vi "Do_Ramsete_SI.vi"(5 "LeftDist-Meters":dbl, 6 "WheelBase-Meters":dbl=2.0, 7 "RightDist-Meters":dbl, 8 "Ramsete Enable":bool, 9 "Path Sample":T4, 10 "Reset":bool, 11 "Gyro-Radians":dbl) -> (0 "AtReference":bool, 1 "RightVelDmd":dbl, 2 "LeftVelDmd":dbl, 3 "CurrentRelativePose":T1, 4 "Err Pose":T1)   [LabVIEW 2019, in "PathExecution_Library.lvlib"]
uses:
  PathExecution_Library.lvlib
  PATH_SAMPLE.ctl
  POSE.ctl
  TRANSLATION.ctl
  ROTATION.ctl
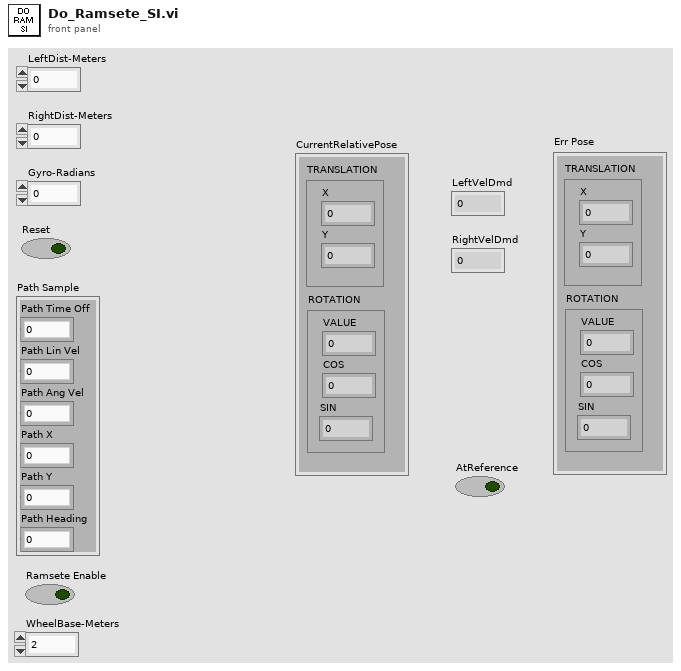
[diagram p1: front panel]
types:
  T1 = typedef "PathExecution_Library.lvlib/POSE.ctl" = cluster{"TRANSLATION":T2, "ROTATION":T3}
  T2 = typedef "PathExecution_Library.lvlib/TRANSLATION.ctl" = cluster{"X":dbl, "Y":dbl}
  T3 = typedef "PathExecution_Library.lvlib/ROTATION.ctl" = cluster{"VALUE":dbl, "COS":dbl, "SIN":dbl}
  T4 = typedef "PathExecution_Library.lvlib/PATH_SAMPLE.ctl" = cluster{"Path Lin Vel":dbl, "Path Ang Vel":dbl, "Path X":dbl, "Path Y":dbl, "Path Heading":dbl, "Path Time Off":dbl}
  T5 = typedef "PathExecution_Library.lvlib/CHASSIS.ctl" = cluster{"vX":dbl, "vY":dbl, "vOmega":dbl}
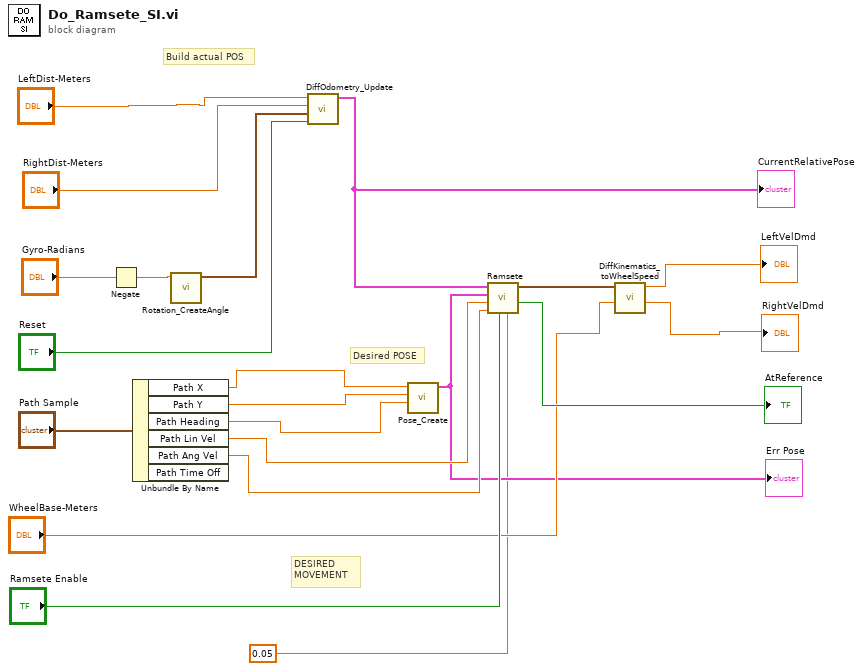
[diagram p0: block diagram]
diagram:
  # "DESIRED\nMOVEMENT"
  # "Desired POSE"
  # "Build actual POS"
  n1 = Negate(x="Gyro-Radians") -> (-x=w3:dbl)
  n2 = Unbundle By Name("Path Sample") -> ("Path X"=w13:dbl, "Path Y"=w12:dbl, "Path Heading"=w11:dbl, "Path Lin Vel"=w10:dbl, "Path Ang Vel"=w9:dbl)  [unwired: 1 out]
  n3 = call "Rotation_CreateAngle.vi"("Angle"=w3) -> ("ROTATION"=w2:T3)  [unwired: 10 in]
  n4 = call "DiffOdometry_Update.vi"("Reset"="Reset", "Heading"=w2, "RightDistance"="RightDist-Meters", "LeftDistance"="LeftDist-Meters") -> ("CurrentRelativePose"=w18:T1)  [unwired: 7 in]
  "CurrentRelativePose" <- w18
  n5 = call "Pose_Create.vi"("Heading"=w11, "Y"=w12, "X"=w13) -> ("out POSe"=w5:T1)  [unwired: 8 in]
  "Err Pose" <- w5
  n6 = call "Ramsete.vi"("POSE TOL"=0.05, "Enabled"="Ramsete Enable", "DesiredAngularVelocity"=w9, "DesiredLinearVelocity"=w10, "DesiredPOSE"=w5, "CurrentPOSE"=w18) -> ("AtReference"=→"AtReference":bool, "CHASSIS Speeds"=w16:T5)  [unwired: 3 in, 1 out]
  n7 = call "DiffKinematics_toWheelSpeed.vi"("TrackWidth_Meters"="WheelBase-Meters", "CHASSIS Speed"=w16) -> ("RightVelocity"=→"RightVelDmd":dbl, "LeftVelocity"=→"LeftVelDmd":dbl)  [unwired: 8 in]
